vi "destroyTCV.vi"(8 "error in (no error)":errorcluster, 11 "ocr in":refnum<class "ocr.lvclass">) -> (0 "error out":errorcluster, 3 "ocr out":refnum<class "ocr.lvclass">)   [LabVIEW 2025, in "adsOCR.lvlib" / "ocr.lvclass"]
uses:
  ocr.lvclass
  ocr.lvclass/ocr.ctl
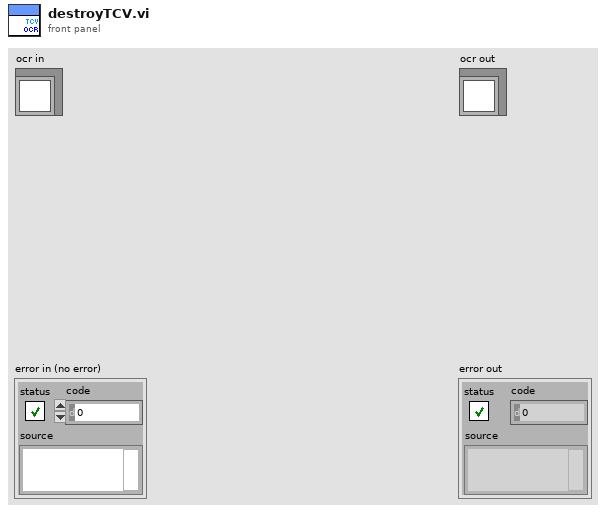
[diagram p1: front panel]
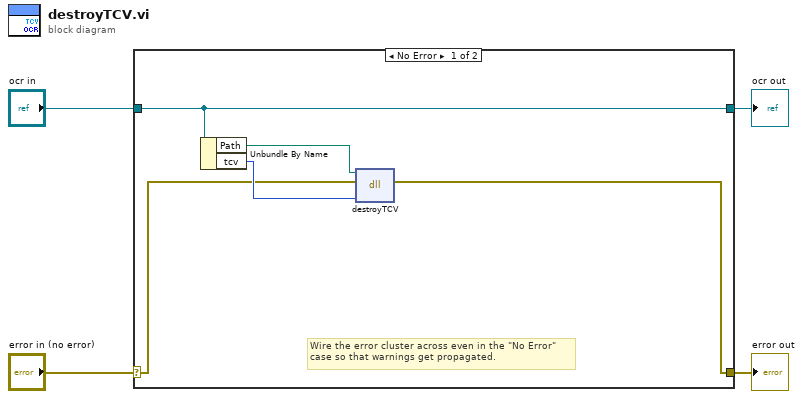
[diagram p0: block diagram]
diagram:
  n1 = case shown="No Error" "error in (no error)" {
    selector: "error in (no error)" -> [w6 w11]
    tunnel: [w5 w11] -> w3
    tunnel: [w9 w10] -> w1
    tunnel: "ocr in" -> [w9 w10]
    frame No Error {
      # "Wire the error cluster across even in the \"No Error\"\ncase so that warnings get propagated."
      n2 = Unbundle By Name(w9) -> ("Path"=w8:path, "tcv"=w7:u64)
      n3 = dll-call lib="D:/Test/adslvPackageDev/Resources/TCV_Lib.dll" fn="destroyTCV"(path in=w8, error in=w6, "tcv"=w7) -> (error out=w5:errorcluster)  [unwired: 3 in, 1 out]
    }
    frame Error {
    }
  }
  "error out" <- w3
  "ocr out" <- w1
